vi "loadGlobal.vi"() -> ()   [LabVIEW 2018]
uses:
  #include/Global_usbComm.vi
panel:
  in  "Sheet#":i32
  in  "pic":bool
  in  "pip":bool=TRUE
  in  "File path":string="C:\\Users\\bryan.lee\\Documents\\GitHub\\LabVIEW\\Projects\\1259_usbComm\\specsheetsConsole\\Documentation\\"
  in  "PIP Instruction Path":path=path "C:/Users/bryan.lee/Documents/GitHub/LabVIEW/Projects/1259_usbComm/specsheetsConsole/Sheets/ConsoleProceduresLabView.xlsx"
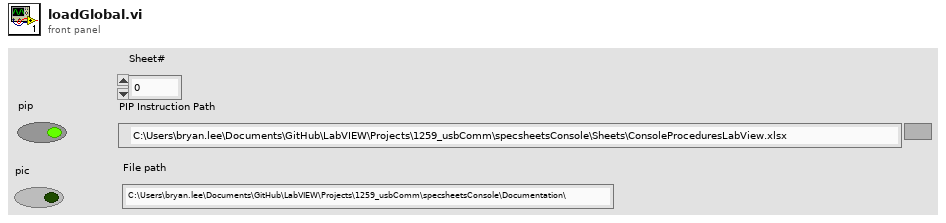
[diagram p1: front panel]
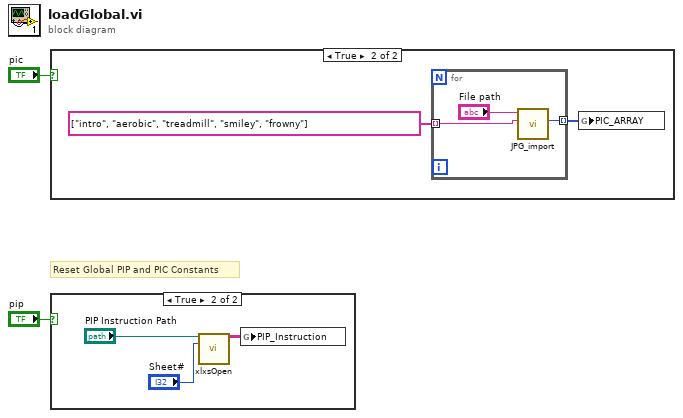
[diagram p0: block diagram]
diagram:
  # "Reset Global PIP and PIC Constants"
  n1 = case shown="True" "pic" {
    frame False {
    }
    frame True {
      n2 = for {
        tunnel: [w6] -> w4 mode=indexing
        tunnel: string[] ["intro", "aerobic", "treadmill", "smiley", "frowny"] -> [w5] mode=indexing
        n3 = call "JPG_import.vi"("File name"=w5, "File path"="File path") -> ("new picture"=w6:picture)  [unwired: 7 in, 2 out]
      }
      n4 = global write "Global_usbComm.vi" "PIC_ARRAY"(w4) -> ()
    }
  }
  n5 = case shown="True" "pip" {
    frame False {
    }
    frame True {
      n6 = call "xlxsOpen.vi"("PIP Instruction Path"="PIP Instruction Path", "Sheet#"="Sheet#") -> ("Shared_strings"=w10:string[][])  [unwired: 9 in, 4 out]
      n7 = global write "Global_usbComm.vi" "PIP_Instruction"(w10) -> ()
    }
  }
